vi "Find Pipette.vi"(0 "Scanning Parameters":T2, 5 "Indicators":T1, 7 "Objects":refnum<vi>, 11 "error in (no error)":errorcluster, 13 "Indicator":refnum<vi>, 14 "Abort ref":refnum<vi>) -> (6 "Pipette Found":bool, 15 "error out":errorcluster)   [LabVIEW 2012, in "Visual Analyser.lvlib"]
uses:
  Visual Analyser.lvlib
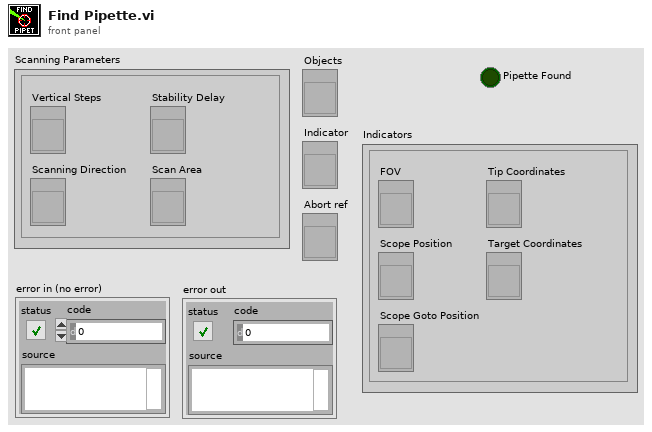
[diagram p1: front panel]
types:
  T1 = cluster{"Tip Coordinates":refnum<vi>, "Target Coordinates":refnum<vi>, "Scope Position":refnum<vi>, "FOV":refnum<vi>, "Scope Goto Position":refnum<vi>}
  T2 = cluster{"Vertical Steps":refnum<vi>, "Stability Delay":refnum<vi>, "Scanning Direction":refnum<vi>, "Scan Area":refnum<vi>}
  T3 = cluster{"X [um]":dbl, "Y [um]":dbl, "Z [um]":dbl}
  T4 = enum16{"Left Button", "Center Button", "Right Button", "Window Close"}
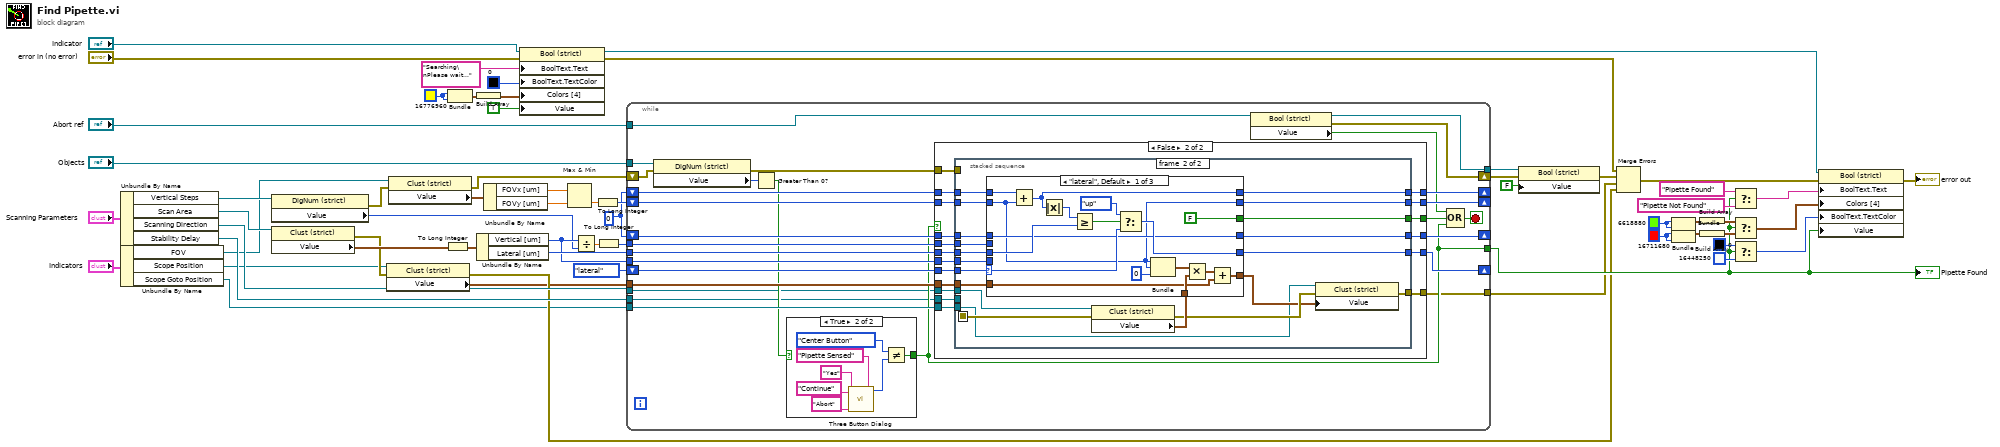
[diagram p0: block diagram]
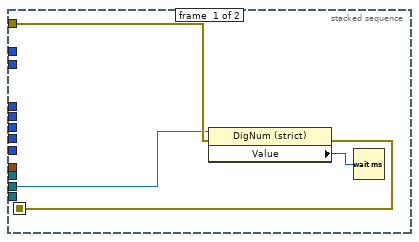
[diagram p3: hidden frame]
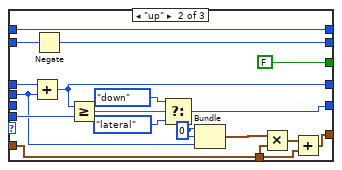
[diagram p4: hidden frame]
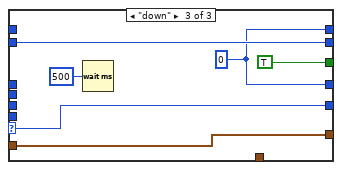
[diagram p5: hidden frame]
diagram:
  w22 = u32 16776960
  w37 = u32 16711680
  w35 = u32 6618880
  w48 = 0
  n1 = Unbundle By Name("Scanning Parameters") -> ("Vertical Steps"=w12:refnum<vi>, "Scan Area"=w9:refnum<vi>, "Scanning Direction"=w10:refnum<vi>, "Stability Delay"=w11:refnum<vi>)
  n2 = Unbundle By Name("Indicators") -> ("FOV"=w1:refnum<vi>, "Scope Position"=w2:refnum<vi>, "Scope Goto Position"=w3:refnum<vi>)
  n3 = property on="Property Node" class="DigNum (strict)"(reference=w12) -> (error out=w14:errorcluster, "Value"=w15:u32)  [unwired: 1 in, 1 out]
  n4 = property on="Property Node" class="Clust (strict)"(reference=w9) -> (error out=w8:errorcluster, "Value"=w16:cluster{"Lateral [um]":dbl, "Vertical [um]":dbl})  [unwired: 1 in, 1 out]
  n5 = property on="Property Node" class="Clust (strict)"(reference=w2, error in=w8) -> (error out=w7:errorcluster, "Value"=w6:T3)  [unwired: 1 out]
  n6 = property on="Property Node" class="Clust (strict)"(reference=w1, error in=w14) -> (error out=w58:errorcluster, "Value"=w49:cluster{"FOVx [um]":dbl, "FOVy [um]":dbl})  [unwired: 1 out]
  n7 = To Long Integer(number=w16) -> (32bit integer=w46:cluster{"Lateral [um]":i32, "Vertical [um]":i32})
  n8 = Bundle(w22, w22) -> (w23:cluster{u32, u32})  [unwired: 1 in]
  n9 = Build Array(w23) -> (w21:cluster{u32, u32}[])
  n10 = Unbundle By Name(w46) -> ("Vertical [um]"=w44:i32, "Lateral [um]"=w55:i32)
  n11 = Unbundle By Name(w49) -> ("FOVx [um]"=w50:dbl, "FOVy [um]"=w51:dbl)
  n12 = property class="Bool (strict)"(reference="Indicator", error in="error in (no error)", "BoolText.Text"="Searching\nPlease wait..." ("Window Title (\"\")"), "BoolText.TextColor"=u32 0, "Colors [4]"=w21, "Value"=TRUE ("Visible")) -> (reference out=w19:refnum<vi>, error out=w20:errorcluster)
  n13 = Max & Min(x=w50, y=w51) -> (min(x,y)=w45:dbl)  [unwired: 1 out]
  n14 = Divide(x=w44, y=w15) -> (x/y=w53:dbl)
  n15 = To Long Integer(number=w45) -> (32bit integer=w52:i32)
  n16 = To Long Integer(number=w53) -> (32bit integer=w54:i32)
  n17 = while {
    shift-right: [w88] -> _
    shift-left: enum16{"lateral", "up", "down"}."lateral" ("Direction") -> [w89]
    tunnel: w54 -> [w87]
    tunnel: w55 -> [w86]
    tunnel: w44 -> [w85]
    shift-right: [w79] -> _
    shift-left: w48 -> [w84]
    shift-right: [w80] -> _
    shift-left: w48 -> [w83]
    shift-right: [w81] -> _
    shift-left: w52 -> [w82]
    tunnel: "Objects" -> [w68]
    tunnel: "Abort ref" -> [w75]
    shift-right: [w74] -> w60
    shift-left: w58 -> [w69]
    tunnel: [w73] -> w61
    tunnel: [w65] -> w27
    tunnel: w3 -> [w72]
    tunnel: w6 -> [w71]
    tunnel: [w64] -> w17
    tunnel: w10 -> [w63]
    tunnel: w11 -> [w62]
    stop <- w78 stop-if-true
    n18 = property on="Property Node" class="DigNum (strict)"(reference=w68, error in=w69) -> (error out=w66:errorcluster, "Value"=w70:i32)  [unwired: 1 out]
    n19 = Greater Than 0?(x=w70) -> (x > 0?=w67:bool)
    n20 = case shown="True" w67 {
      selector: w67 -> [w179 _]
      tunnel: [w179 w180] -> w65
      frame False {
      }
      frame True {
        n21 = call <vilib>:"Three Button Dialog.vi"("Right Button Text (\"Cancel\")"="Abort" ("Right Button Text (\"Cancel\")"), "Center Button Text (\"No\")"="Continue" ("Center Button Text (\"No\")"), "Left Button Text (\"Yes\")"="Yes" ("Left Button Text (\"Yes\")"), "message"="Pipette Sensed") -> ("Which Button?"=w182:T4)  [unwired: 7 in]
        n22 = Not Equal?(x=T4."Center Button", y=w182) -> (x != y?=w180:bool)
      }
    }
    n23 = case shown="False" w65 {
      selector: w65 -> [w91 _]
      tunnel: w89 -> [w92 w113]
      tunnel: [w92 w112] -> w88
      tunnel: w87 -> [_ w111]
      tunnel: w86 -> [_ w110]
      tunnel: w85 -> [_ w109]
      tunnel: w84 -> [w93 w108]
      tunnel: w83 -> [w95 w107]
      tunnel: w82 -> [w94 w106]
      tunnel: [w94 w105] -> w81
      tunnel: [w95 w104] -> w80
      tunnel: [w93 w103] -> w79
      tunnel: [w91 w102] -> w76
      tunnel: w72 -> [_ w101]
      tunnel: w71 -> [_ w100]
      tunnel: w66 -> [w90 w99]
      tunnel: [w90 w98] -> w64
      tunnel: w63 -> [_ w97]
      tunnel: w62 -> [_ w96]
      frame True {
      }
      frame False {
        n24 = stacked-sequence {
          seq-local: [w115 _] -> [_ w123]
          tunnel: w113 -> [_ w137]
          tunnel: [_ w136] -> w112
          tunnel: w111 -> [_ w135]
          tunnel: w110 -> [_ w134]
          tunnel: w109 -> [_ w133]
          tunnel: w108 -> [_ w132]
          tunnel: [_ w131] -> w102
          tunnel: w107 -> [_ w130]
          tunnel: w106 -> [_ w129]
          tunnel: [_ w128] -> w105
          tunnel: [_ w127] -> w104
          tunnel: [_ w126] -> w103
          tunnel: w99 -> [w116 _]
          tunnel: w101 -> [_ w118]
          tunnel: w100 -> [_ w125]
          tunnel: [_ w121] -> w98
          tunnel: w97 -> [_ w122]
          tunnel: w96 -> [w114 _]
          frame #0 {
            n25 = property on="Property Node" class="DigNum (strict)"(reference=w114, error in=w116) -> (error out=w115:errorcluster, "Value"=w117:u32)  [unwired: 1 out]
            n26 = Wait (ms)(milliseconds to wait=w117) -> ()  [unwired: 1 out]
          }
          frame #1 {
            n27 = property on="Property Node" class="Clust (strict)"(reference=w122, error in=w123) -> (error out=w120:errorcluster, "Value"=w124:cluster{"X":i16, "Y":i16, "Z":i16})  [unwired: 1 out]
            n28 = case shown="\"lateral\", Default" w137 {
              selector: w137 -> [w154 _ w175]
              tunnel: [w153 w171 w175] -> w136
              tunnel: w134 -> [w150 _ _]
              tunnel: w135 -> [_ w160 _]
              tunnel: [w144 w166 w176] -> w126
              tunnel: w132 -> [w144 w169 _]
              tunnel: w133 -> [_ w168 _]
              tunnel: [FALSE FALSE TRUE] -> w131
              tunnel: w130 -> [w148 w164 _]
              tunnel: [w145 w164 w176] -> w127
              tunnel: w129 -> [w143 w163 w177]
              tunnel: [w143 w162 w177] -> w128
              tunnel: [w140 w157 w174] -> w119
              tunnel: w124 -> [w141 w158 _]
              tunnel: w125 -> [w138 w155 w174]
              frame "lateral", Default {
                n29 = Add(x=w148, y=w143) -> (x+y=w145:i32)
                n30 = Absolute Value(x=w145) -> (abs(x)=w146:i32)
                n31 = Greater Or Equal?(x=w146, y=w150) -> (x >= y?=w147:bool)
                n32 = Select(t=enum16{"lateral", "up", "down"}."up" ("Direction"), s=w147, f=w154) -> (s? t:f=w153:enum16{"lateral", "up", "down"})
                n33 = Bundle(w143, w143, 0) -> (w142:cluster{i32, i32, i32})  [unwired: 1 in]
                n34 = Multiply(x=w142, y=w141) -> (x*y=w139:cluster{i32, i32, i32})
                n35 = Add(x=w139, y=w138) -> (x+y=w140:cluster{dbl, dbl, dbl})
              }
              frame "up" {
                w161 = 0
                n36 = Add(x=w169, y=w160) -> (x+y=w166:i32)
                n37 = Negate(x=w163) -> (-x=w162:i32)
                n38 = Greater Or Equal?(x=w166, y=w168) -> (x >= y?=w172:bool)
                n39 = Select(t=enum16{"lateral", "up", "down"}."down" ("Direction"), s=w172, f=enum16{"lateral", "up", "down"}."lateral" ("Direction")) -> (s? t:f=w171:enum16{"lateral", "up", "down"})
                n40 = Bundle(w161, w161, w160) -> (w159:cluster{i32, i32, i32})  [unwired: 1 in]
                n41 = Multiply(x=w159, y=w158) -> (x*y=w156:cluster{i32, i32, i32})
                n42 = Add(x=w156, y=w155) -> (x+y=w157:cluster{dbl, dbl, dbl})
              }
              frame "down" {
                w176 = 0
                n43 = Wait (ms)(milliseconds to wait=u32 500) -> ()  [unwired: 1 out]
              }
            }
            n44 = property on="Property Node" class="Clust (strict)"(reference=w118, error in=w120, "Value"=w119) -> (error out=w121:errorcluster)  [unwired: 1 out]
          }
        }
      }
    }
    n45 = property on="Property Node" class="Bool (strict)"(reference=w75) -> (reference out=w73:refnum<vi>, error out=w74:errorcluster, "Value"=w77:bool)  [unwired: 1 in]
    n46 = Compound Arithmetic op=OR(w77, w76, w65) -> (w78:bool)
  }
  "Pipette Found" <- w27
  n47 = property on="Property Node" class="Bool (strict)"(reference=w61, error in=w60, "Value"=FALSE) -> (error out=w29:errorcluster)  [unwired: 1 out]
  n48 = Merge Errors(w20, w29, w17, w7) -> (w28:errorcluster)
  n49 = Bundle(w35, w35) -> (w36:cluster{u32, u32})  [unwired: 1 in]
  n50 = Bundle(w37, w37) -> (w38:cluster{u32, u32})  [unwired: 1 in]
  n51 = Build Array(w36) -> (w33:cluster{u32, u32}[])
  n52 = Build Array(w38) -> (w39:cluster{u32, u32}[])
  n53 = Select(t="Pipette Found" ("Boolean Text.Text"), s=w27, f="Pipette Not Found" ("Window Title (\"\")")) -> (s? t:f=w32:string)
  n54 = Select(t=w33, s=w27, f=w39) -> (s? t:f=w40:cluster{u32, u32}[])
  n55 = Select(t=u32 0, s=w27, f=u32 16448250) -> (s? t:f=w43:u32)
  n56 = property class="Bool (strict)"(reference=w19, error in=w28, "BoolText.Text"=w32, "Colors [4]"=w40, "BoolText.TextColor"=w43, "Value"=w27) -> (error out=→"error out":errorcluster)  [unwired: 1 out]
